vi "Get Heat Control Data.vi"(0 "GEA2 Reference In":refnum<k24>, 11 "Error In":errorcluster) -> (3 "Heat Control Out":T1, 4 "GEA2 Reference Out":refnum<k24>, 15 "Error Out":errorcluster)   [LabVIEW 2016]
uses:
  Tools/Laundry/JL Dryer Tool/JL Dryer Tool Support/type defs/Heat Control.ctl
  Q:/Common/DLLs/GEA3/GeaCommunication.dll
  Common/DLLs/GEA3/GeaCommunication.dll
  Common/LabVIEW GEA2 Toolkit/LabVIEW_GEA2_Toolkit.lvlibp/type defs/ERD Read Data In.ctl
  Common/LabVIEW GEA2 Toolkit/LabVIEW_GEA2_Toolkit.lvlibp/type defs/Data Type.ctl
  Common/LabVIEW GEA2 Toolkit/LabVIEW_GEA2_Toolkit.lvlibp/type defs/Source_Destination.ctl
  Common/LabVIEW GEA2 Toolkit/LabVIEW_GEA2_Toolkit.lvlibp
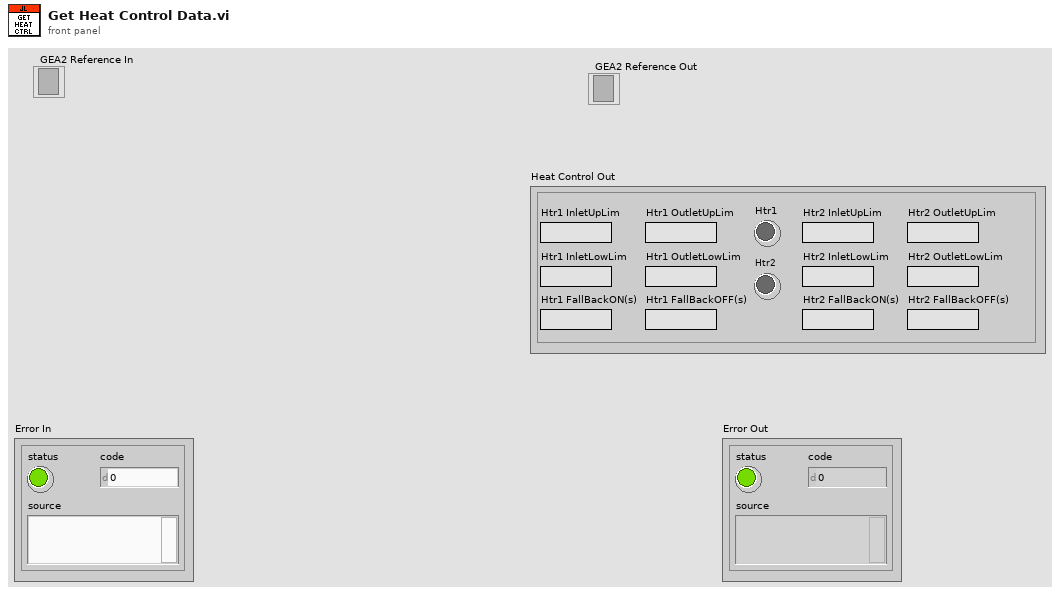
[diagram p1: front panel]
types:
  T1 = typedef "Heat Control.ctl" = cluster{"Htr1 InletLowLim":string, "Htr1 InletUpLim":string, "Htr1 OutletLowLim":string, "Htr1 OutletUpLim":string, "Htr1 FallBackON(s)":string, "Htr1 FallBackOFF(s)":string, "Htr1":bool, "Htr2 InletLowLim":string, "Htr2 InletUpLim":string, "Htr2 OutletLowLim":string, "Htr2 OutletUpLim":string, "Htr2 FallBackON(s)":string, "Htr2 FallBackOFF(s)":string, "Htr2":bool}
  T2 = typedef "LabVIEW_GEA2_Toolkit.lvlibp/Source_Destination.ctl" = cluster{"Source":u8, "Destination":u8}
  T3 = typedef "LabVIEW_GEA2_Toolkit.lvlibp/ERD Read Data In.ctl" = cluster{"ERD Number":u16, "Data Type":T4}
  T4 = typedef "LabVIEW_GEA2_Toolkit.lvlibp/Data Type.ctl" = enum16{"string", "boolean", "uint8_t", "uint16_t", "uint32_t", "uint64_t", "int8_t", "int16_t", "int32_t", "int64_t"}
  T5 = typedef "LabVIEW_GEA2_Toolkit.lvlibp/ERD Read Data Out.ctl" = cluster{"ERD Number":u16, "Data":string}
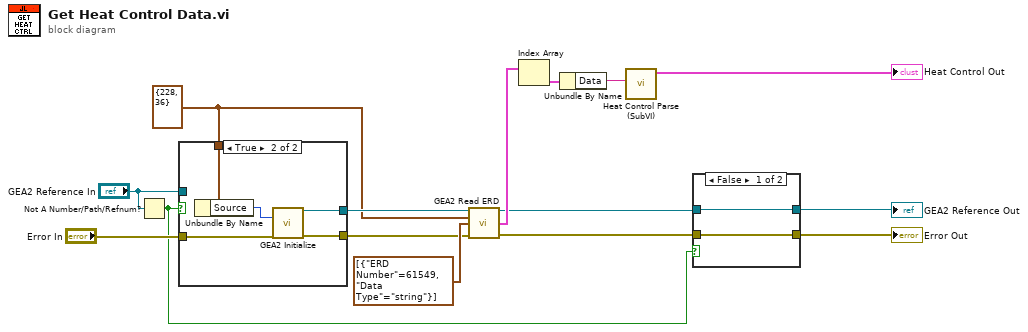
[diagram p0: block diagram]
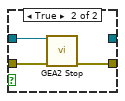
[diagram p2: hidden frame]
diagram:
  w7 = T2 {"Source"=228, "Destination"=36} ("GEA Inputs")
  n1 = Not A Number/Path/Refnum?(number/path/refnum="GEA2 Reference In") -> (NaN/Path/Refnum?=w1:bool)
  n2 = case shown="True" w1 {
    tunnel: w7 -> [_ w22]
    tunnel: "GEA2 Reference In" -> [w16 _]
    tunnel: "Error In" -> [w17 w20]
    tunnel: [w16 w19] -> w13
    tunnel: [w17 w18] -> w11
    frame False {
    }
    frame True {
      n3 = Unbundle By Name(w22) -> ("Source"=w21:u8)
      n4 = call "GEA2 Initialize.vi"("Source Address"=w21, "error in"=w20) -> ("GEA2 Reference Out"=w19:refnum<k24>, "error out"=w18:errorcluster)  [unwired: 11 in, 1 out]
    }
  }
  n5 = call "GEA2 Read ERD.vi"("GEA2 Reference In"=w13, "GEA Inputs"=w7, "Read ERD List"=T3[] [{"ERD Number"=61549, "Data Type"=enum."string"}], "Error In"=w11) -> ("GEA2 Reference Out"=w4:refnum<k24>, "ERD Data Out"=w9:T5[], "Error Out"=w5:errorcluster)  [unwired: 8 in, 1 out]
  n6 = Index Array(array=w9) -> (element=w10:T5)  [unwired: 1 in]
  n7 = Unbundle By Name(w10) -> ("Data"=w8:string)
  n8 = call "Heat Control Parse (SubVI).vi"("Data"=w8) -> ("Heat Control out"=→"Heat Control Out":T1)  [unwired: 10 in]
  n9 = case shown="False" w1 {
    tunnel: [w23 w27] -> w6
    tunnel: w4 -> [w24 w26]
    tunnel: [w24 _] -> w3
    tunnel: w5 -> [w23 w25]
    frame False {
    }
    frame True {
      n10 = call "GEA2 Stop.vi"("GEA2 Reference In"=w26, "Error In"=w25) -> ("Error Out"=w27:errorcluster)  [unwired: 13 in]
    }
  }
  "Error Out" <- w6
  "GEA2 Reference Out" <- w3
